vi "attribute_write_string.vi"(5 "Repeated Capability":string, 7 "Attribute":T1={"Identifier"="", "Descriptive name"="", "Data Type"=enum."Integer 32", "Command"="", "Access"=2, "Range Table"="", "Read Callback"="", "Write Callback"="", "Range Callback"="", "Check Callback"="", "Rngtable Callback"="", "Coerce Callback"="", "Supported Models"="", "Instrument Options"="", "Repeated Capabilities"="", "Check Status Callback"="", "Index"=0, "Flag: OPC Wait"=FALSE, "Flag: Dont check status"=FALSE, "Flag: Cache Only"=FALSE} {"Access" items=["Read Only", "Write Only", "Read/Write"]}, 8 "error in":errorcluster, 10 "string in":string, 11 "VISA resource name":refnum<visa-resource-name>) -> (0 "error out":errorcluster, 3 "VISA resource name out":refnum<visa-resource-name>)   [LabVIEW 2014, in "rszvl_rsidr_core.lvlib"]
uses:
  rszvl_rsidr_core.lvlib
  type_Attribute.ctl
  type_Attribute_Data_Type.ctl
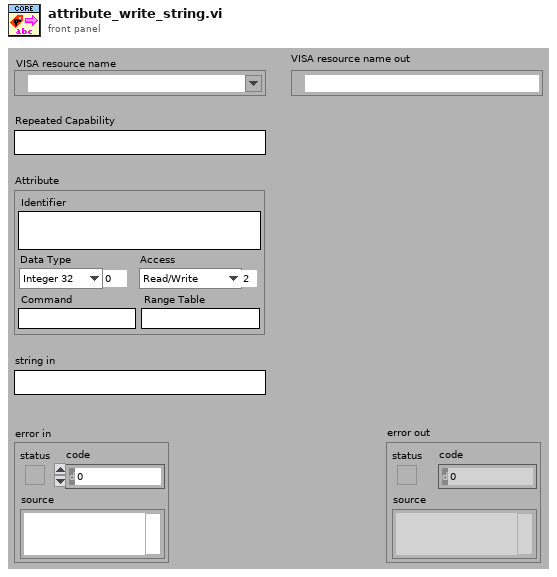
[diagram p1: front panel]
types:
  T1 = typedef "rszvl_rsidr_core.lvlib/type_Attribute.ctl" = cluster{"Identifier":string, "Descriptive name":string, "Data Type":T2, "Command":string, "Access":u16, "Range Table":string, "Read Callback":string, "Write Callback":string, "Range Callback":string, "Check Callback":string, "Rngtable Callback":string, "Coerce Callback":string, "Supported Models":string, "Instrument Options":string, "Repeated Capabilities":string, "Check Status Callback":string, "Index":i32, "Flag: OPC Wait":bool, "Flag: Dont check status":bool, "Flag: Cache Only":bool}
  T2 = typedef "rszvl_rsidr_core.lvlib/type_Attribute_Data_Type.ctl" = enum16{"Integer 32", "Double", "String", "Boolean", "None", "Integer 64"}
  T3 = typedef "rszvl_rsidr_core.lvlib/type_Session_Data.ctl" = cluster{"Instr type":string, "Instr type for err. msg.":string, "Installed Options":string[], "OPC Timeout":i32, "Query Instrument Status":bool, "Check Range":bool, "Check Options":bool, "Add LF to Write":bool, "Simulate":bool, "Logging":bool, "Logging params":variant, "Interface Type":enum16{"Unknown", "GPIB", "VXI", "GPIB_VXI", "ASRL", "PXI", "TCPIP", "USB", "SOCKET"}, "Fast Sweep":i32, "AdditionalFlags":i32, "WaitBeforeWrite":i32, "WaitBeforeRead":i32, "BinDataChunkSize":i64}
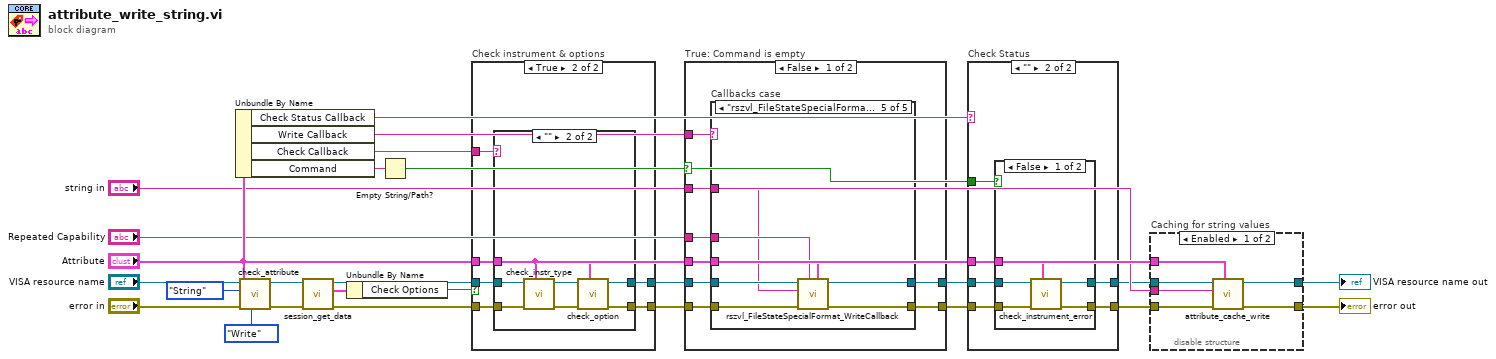
[diagram p0: block diagram]
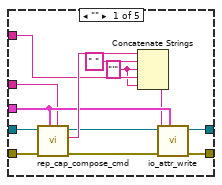
[diagram p2: hidden frame]
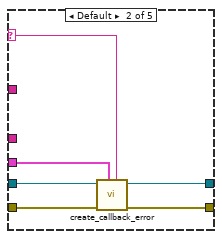
[diagram p3: hidden frame]
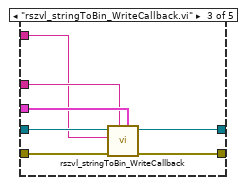
[diagram p4: hidden frame]
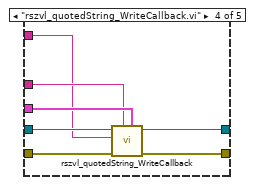
[diagram p5: hidden frame]
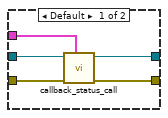
[diagram p7: hidden frame]
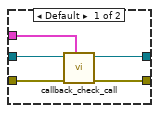
[diagram p10: hidden frame]
diagram:
  n1 = Unbundle By Name("Attribute") -> ("Check Status Callback"=w11:string, "Write Callback"=w15:string, "Check Callback"=w16:string, "Command"=w1:string)
  n2 = call "check_attribute.vi"("Access"=enum16{"Read", "Write"}."Write", "Attribute"="Attribute", "error in"="error in", "Data Type"=type_Attribute_Data_Type."String", "VISA resource name"="VISA resource name") -> ("error out"=w10:errorcluster, "VISA resource name out"=w9:refnum<visa-resource-name>)  [unwired: 5 in]
  n3 = call "session_get_data.vi"("error in"=w10, "VISA resource name"=w9) -> ("error out"=w8:errorcluster, "Session User Data out"=w13:T3, "VISA resource name out"=w7:refnum<visa-resource-name>)  [unwired: 7 in]
  n4 = Unbundle By Name(w13) -> ("Check Options"=w14:bool)
  n5 = Empty String/Path?(string/path=w1) -> (empty?=w26:bool)
  n6 = case "Check instrument & options" shown="True" w14 {
    tunnel: [w28 w29] -> w5
    tunnel: [w27 w30] -> w6
    tunnel: "Attribute" -> [_ w34]
    tunnel: w16 -> [_ w33]
    tunnel: w7 -> [w28 w31]
    tunnel: w8 -> [w27 w32]
    frame False {
    }
    frame True {
      n7 = case shown="\"\"" w33 {
        tunnel: [w38 w41] -> w29
        tunnel: [w36 w42] -> w30
        tunnel: w32 -> [w37 w46]
        tunnel: w34 -> [w35 w40]
        tunnel: w31 -> [w39 w45]
        frame Default {
          n8 = call "callback_check_call.vi"("Attribute"=w35, "error in"=w37, "VISA resource name"=w39) -> ("error out"=w36:errorcluster, "VISA resource name out"=w38:refnum<visa-resource-name>)  [unwired: 7 in]
        }
        frame "" {
          n9 = call "check_instr_type.vi"("Attribute"=w40, "error in"=w46, "VISA resource name"=w45) -> ("error out"=w44:errorcluster, "VISA resource name out"=w43:refnum<visa-resource-name>)  [unwired: 6 in, 1 out]
          n10 = call "check_option.vi"("Attribute"=w40, "error in"=w44, "VISA resource name"=w43) -> ("error out"=w42:errorcluster, "VISA resource name out"=w41:refnum<visa-resource-name>)  [unwired: 7 in]
        }
      }
    }
  }
  n11 = case "True: Command is empty" shown="False" w26 {
    tunnel: "Repeated Capability" -> [w54 _]
    tunnel: w6 -> [w50 w95]
    tunnel: w5 -> [w49 w96]
    tunnel: "string in" -> [w53 _]
    tunnel: "Attribute" -> [w52 _]
    tunnel: [w47 w96] -> w3
    tunnel: [w48 w95] -> w4
    tunnel: w15 -> [w51 _]
    frame False {
      n12 = case "Callbacks case" shown="\"rszvl_FileStateSpecialFormat_WriteCallback.vi\"" w51 {
        selector: w51 -> [_ w68 _ _ _]
        tunnel: w53 -> [w66 _ w76 w83 w90]
        tunnel: w49 -> [w64 w72 w79 w86 w93]
        tunnel: w50 -> [w65 w73 w80 w87 w94]
        tunnel: w54 -> [w58 _ w77 w84 w91]
        tunnel: [w60 w70 w74 w81 w88] -> w47
        tunnel: [w61 w71 w75 w82 w89] -> w48
        tunnel: w52 -> [w59 w69 w78 w85 w92]
        frame "" {
          w56 = "'" ("string")
          n13 = call "rep_cap_compose_cmd.vi"("Repeated Capability"=w58, "Attribute"=w59, "error in"=w65, "VISA resource name"=w64) -> ("error out"=w63:errorcluster, "Command out"=w67:string, "VISA resource name out"=w62:refnum<visa-resource-name>)  [unwired: 5 in]
          n14 = Concatenate Strings(w67, " " ("string"), w56, w66, w56) -> (w55:string)
          n15 = call "io_attr_write.vi"("Attribute"=w59, "error in"=w63, "write buffer"=w55, "VISA resource name"=w62) -> ("error out"=w61:errorcluster, "VISA resource name out"=w60:refnum<visa-resource-name>)  [unwired: 6 in]
        }
        frame Default {
          n16 = call "create_callback_error.vi"("Callback Name"=w68, "Attribute"=w69, "error in"=w73, "VISA resource name"=w72) -> ("error out"=w71:errorcluster, "VISA resource name out"=w70:refnum<visa-resource-name>)  [unwired: 6 in]
        }
        frame "rszvl_stringToBin_WriteCallback.vi" {
          n17 = call "rszvl_stringToBin_WriteCallback.vi"("Attribute"=w78, "Repeated Capability"=w77, "error in"=w80, "Attribute Value String"=w76, "VISA resource name"=w79) -> ("error out"=w75:errorcluster, "VISA resource name out"=w74:refnum<visa-resource-name>)  [unwired: 5 in]
        }
        frame "rszvl_quotedString_WriteCallback.vi" {
          n18 = call "rszvl_quotedString_WriteCallback.vi"("Attribute"=w85, "Repeated Capability"=w84, "error in"=w87, "Attribute Value String"=w83, "VISA resource name"=w86) -> ("error out"=w82:errorcluster, "VISA resource name out"=w81:refnum<visa-resource-name>)  [unwired: 5 in]
        }
        frame "rszvl_FileStateSpecialFormat_WriteCallback.vi" {
          n19 = call "rszvl_FileStateSpecialFormat_WriteCallback.vi"("Attribute"=w92, "Repeated Capability"=w91, "error in"=w94, "Attribute Value String"=w90, "VISA resource name"=w93) -> ("error out"=w89:errorcluster, "VISA resource name out"=w88:refnum<visa-resource-name>)  [unwired: 5 in]
        }
      }
    }
    frame True {
    }
  }
  n20 = case "Check Status" shown="\"\"" w11 {
    tunnel: w4 -> [w101 w105]
    tunnel: [w100 w103] -> w20
    tunnel: [w99 w102] -> w19
    tunnel: w3 -> [w98 w104]
    tunnel: "Attribute" -> [w97 w107]
    tunnel: w26 -> [_ w106]
    frame Default {
      n21 = call "callback_status_call.vi"("Attribute"=w97, "error in"=w101, "VISA resource name"=w98) -> ("error out"=w100:errorcluster, "VISA resource name out"=w99:refnum<visa-resource-name>)  [unwired: 7 in]
    }
    frame "" {
      n22 = case shown="False" w106 {
        tunnel: w104 -> [w111 w114]
        tunnel: w105 -> [w112 w113]
        tunnel: [w110 w113] -> w103
        tunnel: [w109 w114] -> w102
        tunnel: w107 -> [w108 _]
        frame False {
          n23 = call "check_instrument_error.vi"("Attribute"=w108, "error in"=w112, "VISA resource name"=w111) -> ("error out"=w110:errorcluster, "VISA resource name out"=w109:refnum<visa-resource-name>)  [unwired: 7 in]
        }
        frame True {
        }
      }
    }
  }
  n24 = disable-structure "Caching for string values" shown="Enabled" {
    disable-tunnel: [w118 w122] -> w17
    disable-tunnel: [w116 w121] -> w18
    disable-tunnel: w20 -> [w117 w121]
    disable-tunnel: w19 -> [w119 w122]
    disable-tunnel: "string in" -> [w115 _]
    disable-tunnel: "Attribute" -> [w120 _]
    frame Enabled {
      n25 = call "attribute_cache_write.vi"("Attribute"=w120, "error in"=w117, "Value in"=w115, "VISA resource name"=w119) -> ("error out"=w116:errorcluster, "VISA resource name out"=w118:refnum<visa-resource-name>)  [unwired: 6 in]
    }
    frame Disabled {
    }
  }
  "error out" <- w18
  "VISA resource name out" <- w17
